vi "Feb18_2016.vi"(9 "Image 2":T1(plugin-control), 10 "Sequence Storer":T2[][](array[typedef]) {"Amplitude Correction" step=0.1; "Line Trapping"."Phase Gradient" step=0.05; "Line Trapping"."Vector"."x" step=1e-06 format="%#_6p"; "Line Trapping"."Vector"."y" step=1e-06 format="%#_6p"; "Line Trapping"."Vector"."z" step=1e-06 format="%#_6p"; "NA Position"."r" step=1e-06; "NA Position"."y" step=1e-06; "NA Position"."x" step=1e-06; "Position"."z" step=1e-06; "Position"."y" step=1e-06; "Position"."x" step=1e-06; "Phase" step=0.7753; "Intensity" step=0.1}) -> ()   [LabVIEW 2015]
uses:
  subvis/spot.ctl
  subvis/line_trapping.ctl
panel:
  in  "Array":cluster{"x":dbl, "y":dbl}[](array[cluster])
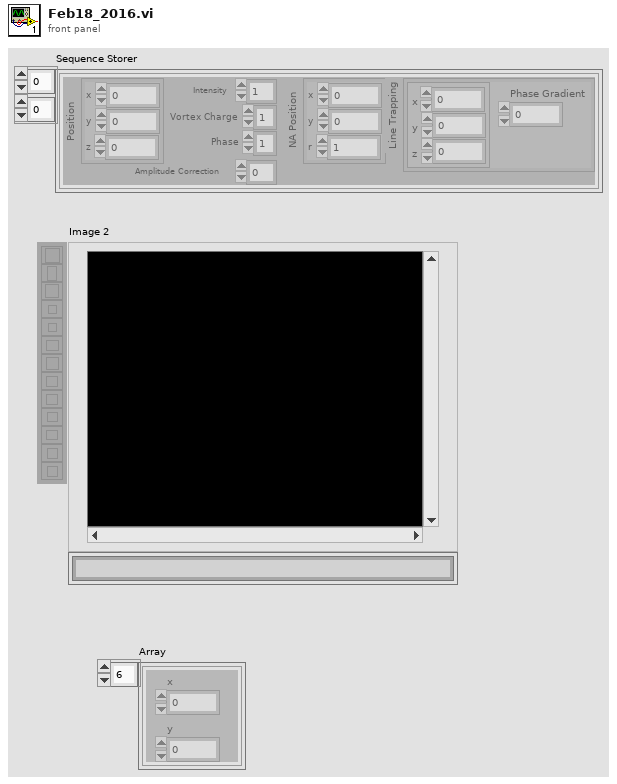
[diagram p1: front panel]
types:
  T1 = typedef "IMAQ Image.ctl" = refnum<image>
  T2 = typedef "spot.ctl" = cluster{"Position":cluster{"x":dbl, "y":dbl, "z":dbl}, "Intensity":dbl, "Vortex Charge":i8, "Phase":dbl, "NA Position":cluster{"x":dbl, "y":dbl, "r":dbl}, "Line Trapping":T3, "Amplitude Correction":dbl}
  T3 = typedef "line_trapping.ctl" = cluster{"Vector":cluster{"x":dbl, "y":dbl, "z":dbl}, "Phase Gradient":dbl}
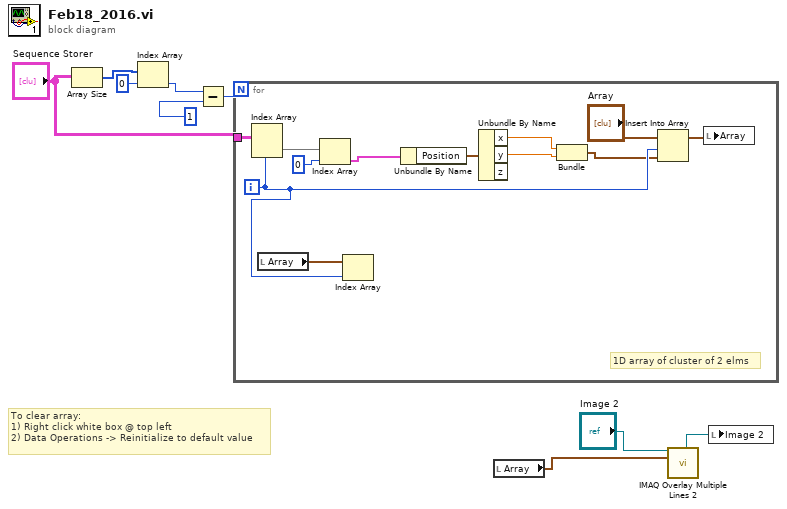
[diagram p0: block diagram]
diagram:
  # "To clear array: \n1) Right click white box @ top left\n2) Data Operations -> Reinitialize to default value"
  n1 = Array Size(array="Sequence Storer") -> (size(s)=w7:i32[])
  n2 = Index Array(array=w7, index=0) -> (element=w6:i32)
  n3 = Subtract(x=w6, y=1) -> (x-y=w5:i32)
  n4 = for {
    N: w5 -> [_]
    tunnel: "Sequence Storer" -> [w21]
    i -> [w13]
    # "1D array of cluster of 2 elms"
    n5 = Index Array(array=w21, index (row)=w13) -> (element=w17:T2[])  [unwired: 1 in]
    n6 = local read "Array"() -> (w11:cluster{"x":dbl, "y":dbl}[])
    n7 = Index Array(array=w17, index=0) -> (element=w15:T2)
    n8 = Index Array(array=w11, index=w13) -> ()  [unwired: 1 out]
    n9 = Unbundle By Name(w15) -> ("Position"=w14:cluster{"x":dbl, "y":dbl, "z":dbl})
    n10 = Unbundle By Name(w14) -> ("x"=w20:dbl, "y"=w19:dbl)  [unwired: 1 out]
    n11 = Bundle("x"=w20, "y"=w19) -> (w10:cluster{"x":dbl, "y":dbl})  [unwired: 1 in]
    n12 = Insert Into Array(array="Array", index=w13, new element=w10) -> (w12:cluster{"x":dbl, "y":dbl}[])
    n13 = local write "Array"(w12) -> ()
  }
  n14 = local read "Array"() -> (w1:cluster{"x":dbl, "y":dbl}[])
  n15 = call "IMAQ Overlay Multiple Lines 2"("Image"="Image 2", "Line End Points"=w1) -> ("Image Out"=w2:T1)  [unwired: 12 in, 1 out]
  n16 = local write "Image 2"(w2) -> ()
